vi "OSSCAR_v3_BM.vi"() -> ()   [LabVIEW 2021]
uses:
  SubVIs/Plot_trap_heating_global_BM.vi
  SubVIs/OSSCAR_stop_global_BM.vi
  SubVIs/DMSO-related/Temp_global_BM.vi
panel:
  out "Current Analyte:":string="DMS"
  in  "N std pt.s":i32=6
  in  "Mode Selection":T1(ring)
  in  "Standalone Function":T2(ring)
  out "Reduction Countdown (min)":dbl format="%.2g"
  out "Hydrolysis Countdown (min)":dbl format="%.2g"
  out "Sparge Countdown (min)":dbl format="%.2g"
  out "Elution Countdown (min)":dbl format="%.2f"
  out "Hydrolysis Progress Bar":u8(slide)=100 scale=0.0..100.0
  out "Reduction Progress Bar":u8(slide)=100 scale=0.0..100.0
  out "Elution Progress Bar":u8(slide)=100 scale=0.0..100.0
  out "Sparging Progress Bar":u8(slide)=100 scale=0.0..100.0
  in  "Analysis Type":T3(ring)
  in  "Tab Control":T4(tab)
  in  "Metadata":T5={"Local save location:"="C:\\Users\\LabPC1\\OneDrive\\Desktop\\OSSCAR_metadata\\Test_metadata", "Cruise ID"="LaPerouse", "Sampling Timestamp"="2023-07-19 15:23:13", "Elution Timestamp"="2023-07-19 15:29:12", "GPS_Latitude"=-999.0, "GPS_Longitude"=-999.0, "DMS_std_conc"=0.0, "DMSP_std_conc"=0.0, "DMSO_std_conc"=0.0, "Std_index"=0.0, "Initial Trap Temp (oC)"=30.0, "Max Trap Temp (oC)"=304.0, "Final Trap Temp (oC)"=30.0, "Flow Rate (mL/min)"=0.0, "Comment"="", "GPS_Minute"=-999.0, "GPS_Day"=-999.0, "GPS_jd"=-999.0, "GPS_Hour"=-999.0, "GPS_Second"=-999.0, "GPS Baud"=4800.0, "COM Port (GPS)"="COM10", "Use GPS?"=FALSE, "Format Date"="%d-%d-%d"} {"GPS_Latitude" format="%_4g"; "GPS_Longitude" format="%_4g"; "GPS_jd" format="%_5g"; "Std_index" format="%.2g"; "DMSO_std_conc" format="%.2f"; "DMSP_std_conc" format="%.2f"; "DMS_std_conc" format="%.2f"}
  in  "Sample Params":T6={"DMS Sparge Time (min)"=7.0, "Elution Time (min)"=1.5, "COM port (16 Pos. Valve)"="COM10", "Trap Heating Time (ms)"=500.0, "COM Port (DC Power)"="COM5", "COM Port (Runze)"="COM3", "sample volume"=10.0, "DMSO red. Sparge Time  (min)"=32.0, "DMSO Red. Duration (min)"=30.0, "Bypass sample handling (debugging)"=FALSE, "Reverse Reduction?"=FALSE, "Voltage (V)"="4.0", "DMSP Hydrolysis Time (min)"=13.0}
  in  "Constants":T7={"step to ml"=1920.0, "BoardNum"=0, "PosA BitNum"=1, "PosB BitNum"=2, "Heat Pulse Delay (ms)"=1000.0, "Heating Iterations"=6, "N rinses"=2, "Dissolution Time (s)"=120, "SpargeBit"=0, "Extra Milli-Q (ml)"=2.0, "Valco Port Number"=6, "BitNum (Thermocouple)"=1, "Total Vol. (mL)"=10.0, "N syringe rinses"=2, "NaOH Vol (ml)"=2.0, "FanBit"=4}
  in  "Pump Parameters":T8={"Speed 1"="100", "Speed 2"="250", "Speed 3"="350", "Speed 4"="250", "UW/Sample"="5", "Sparge"="2", "Std"="4", "Waste"="15", "Air"="14", "Milli-Q"="1", "H2SO4"="6", "NaOH"="3", "Catalyst"="7", "Cell (H+ side)"="8", "Cell (sample side)"="9", "NaCl"="11"}
  out "Current Temp:":i32=29
  out "Trap Heating":cluster{"Y":dbl[], "Y":dbl[]}[](graph)
  # "OSSCAR DMS/O/P Program"
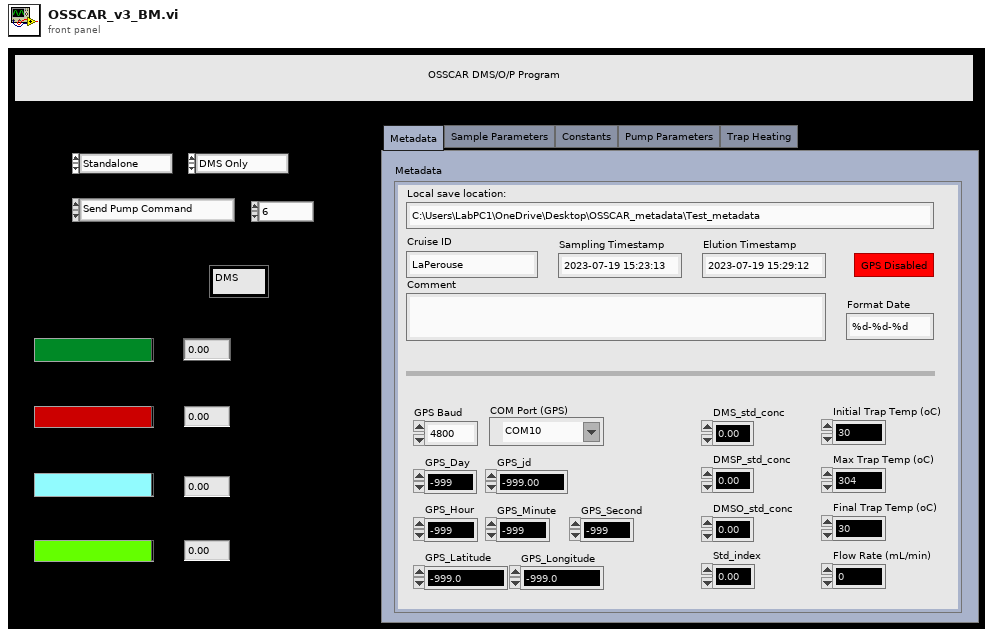
[diagram p1: front panel]
types:
  T1 = enum16{"Standalone", "Analysis", "Standard Curve", "Point Std"}
  T2 = enum16{"Send Pump Command", "Condition Trap", "Control Fan", "Control Sparger", "Load/Inject Trap", "Switch Flow Path", "Control cell DC power", "Rinse Sparge Chamber", "Rinse Cell"}
  T3 = enum16{"DMS Only", "DMS/O", "DMS/P", "DMS/O/P", "DMSO Only"}
  T4 = enum32{"Metadata", "Sample Parameters", "Constants", "Pump Parameters", "Trap Heating"}
  T5 = cluster{"Local save location:":string, "Cruise ID":string, "Sampling Timestamp":string, "Elution Timestamp":string, "GPS_Latitude":dbl, "GPS_Longitude":dbl, "DMS_std_conc":dbl, "DMSP_std_conc":dbl, "DMSO_std_conc":dbl, "Std_index":dbl, "Initial Trap Temp (oC)":dbl, "Max Trap Temp (oC)":dbl, "Final Trap Temp (oC)":dbl, "Flow Rate (mL/min)":dbl, "Comment":string, "GPS_Minute":dbl, "GPS_Day":dbl, "GPS_jd":dbl, "GPS_Hour":dbl, "GPS_Second":dbl, "GPS Baud":dbl, "COM Port (GPS)":refnum<visa-resource-name>, "Use GPS?":bool, "Format Date":string}
  T6 = cluster{"DMS Sparge Time (min)":dbl, "Elution Time (min)":dbl, "COM port (16 Pos. Valve)":refnum<visa-resource-name>, "Trap Heating Time (ms)":dbl, "COM Port (DC Power)":refnum<visa-resource-name>, "COM Port (Runze)":refnum<visa-resource-name>, "sample volume":dbl, "DMSO red. Sparge Time  (min)":dbl, "DMSO Red. Duration (min)":dbl, "Bypass sample handling (debugging)":bool, "Reverse Reduction?":bool, "Voltage (V)":string, "DMSP Hydrolysis Time (min)":dbl}
  T7 = cluster{"step to ml":dbl, "BoardNum":u32, "PosA BitNum":u32, "PosB BitNum":u32, "Heat Pulse Delay (ms)":dbl, "Heating Iterations":i32, "N rinses":i32, "Dissolution Time (s)":u32, "SpargeBit":u32, "Extra Milli-Q (ml)":dbl, "Valco Port Number":i32, "BitNum (Thermocouple)":u32, "Total Vol. (mL)":dbl, "N syringe rinses":i32, "NaOH Vol (ml)":dbl, "FanBit":u32}
  T8 = cluster{"Speed 1":string, "Speed 2":string, "Speed 3":string, "Speed 4":string, "UW/Sample":string, "Sparge":string, "Std":string, "Waste":string, "Air":string, "Milli-Q":string, "H2SO4":string, "NaOH":string, "Catalyst":string, "Cell (H+ side)":string, "Cell (sample side)":string, "NaCl":string}
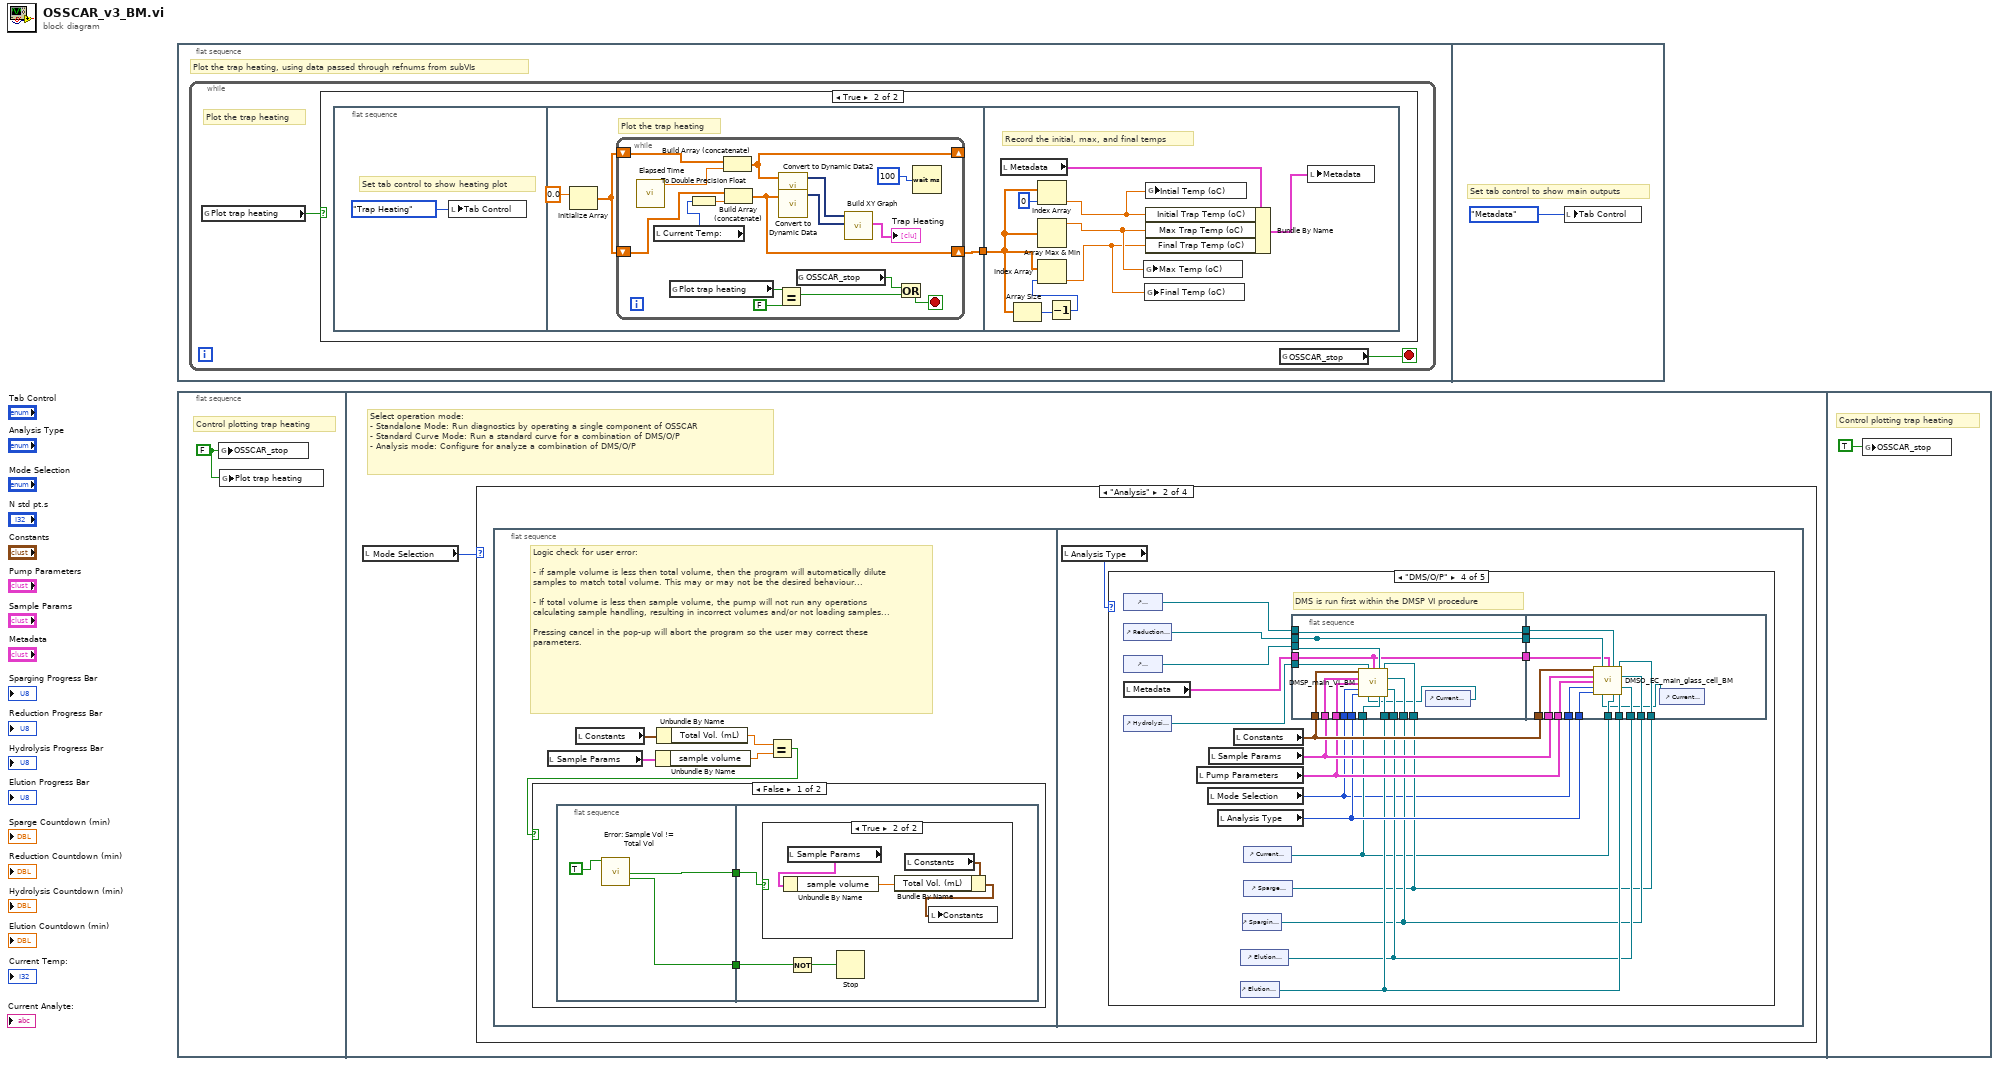
[diagram p0: block diagram]
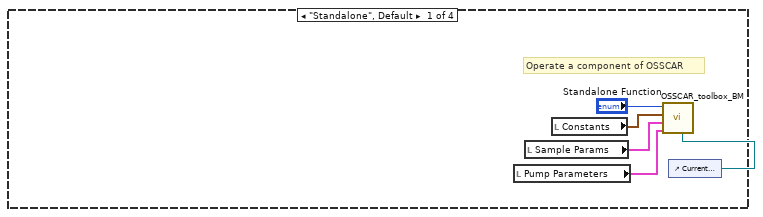
[diagram p3: hidden frame]
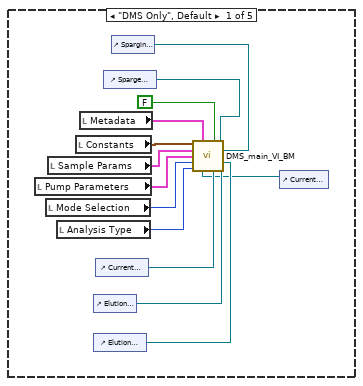
[diagram p6: hidden frame]
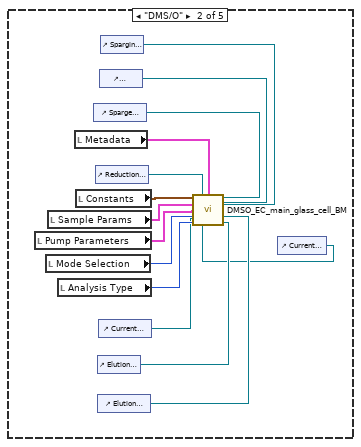
[diagram p7: hidden frame]
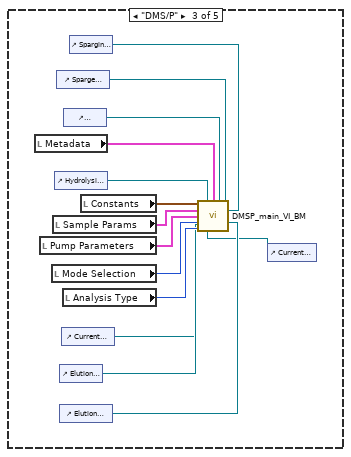
[diagram p8: hidden frame]
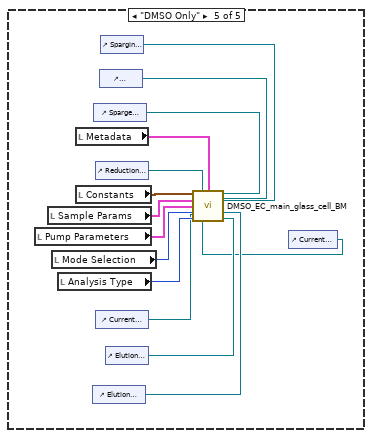
[diagram p9: hidden frame]
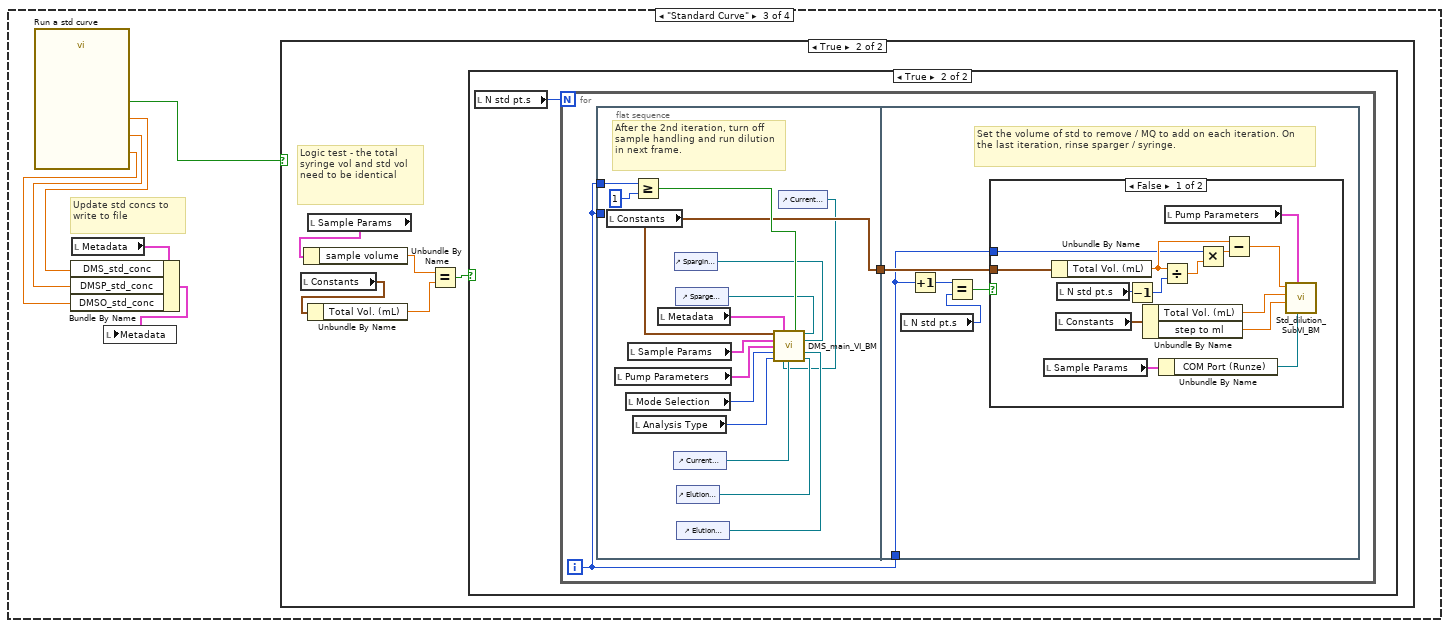
[diagram p10: hidden frame]
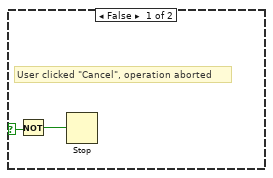
[diagram p11: hidden frame]
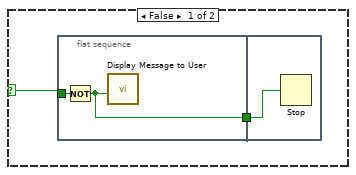
[diagram p12: hidden frame]
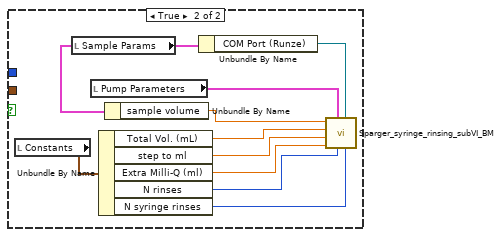
[diagram p13: hidden frame]
diagram:
  n1 = flat-sequence {
    frame #0 {
      # "Plot the trap heating, using data passed through refnums from subVIs"
      n2 = while {
        stop <- w2 stop-if-true
        # "Plot the trap heating"
        n3 = global read "Plot_trap_heating_global_BM.vi" "Plot trap heating"() -> (w1:bool)
        n4 = case shown="True" w1 {
          frame False {
            # "Do nothing when the trap isn't heating"
          }
          frame True {
            n5 = flat-sequence {
              tunnel: [w7] -> w3
              tunnel: w3 -> [w27]
              frame #0 {
                # "Set tab control to show heating plot"
                n6 = local write "Tab Control"(T4."Trap Heating" ("Tab Control 2")) -> ()
              }
              frame #1 {
                # "Plot the trap heating"
                n7 = Initialize Array(0.0 ("element")) -> (w5:dbl[])  [unwired: 1 in]
                n8 = while {
                  shift-right: [w14] -> w7
                  shift-left: w5 -> [w16]
                  shift-right: [w9] -> _
                  shift-left: w5 -> [w11]
                  stop <- w21 stop-if-true
                  n9 = call "Elapsed Time"() -> ("Elapsed Time (s)"=w12:dbl)  [unwired: 12 in, 7 out]
                  n10 = local read "Current Temp:"() -> (w23:i32)
                  n11 = global read "Plot_trap_heating_global_BM.vi" "Plot trap heating"() -> (w20:bool)
                  n12 = To Double Precision Float(number=w23) -> (double precision float=w17:dbl)
                  n13 = Build Array (concatenate)(w11, w12) -> (w9:dbl[])
                  n14 = Build Array (concatenate)(w16, w17) -> (w14:dbl[])
                  n15 = Equal?(x=w20, y=FALSE) -> (x = y?=w18:bool)
                  n16 = call "Convert to Dynamic Data2"("Array"=w9) -> ("Dynamic Data Type"=w10:dynamicdata)  [unwired: 3 in]
                  n17 = call "Convert to Dynamic Data"("Array"=w14) -> ("Dynamic Data Type"=w13:dynamicdata)  [unwired: 3 in]
                  n18 = global read "OSSCAR_stop_global_BM.vi" "OSSCAR_stop"() -> (w22:bool)
                  n19 = call "Build XY Graph"("Y Input"=w13, "X Input"=w10) -> ("XY Graph"=→"Trap Heating":cluster{"X":dbl[], "Y":dbl[]}[])  [unwired: 8 in, 1 out]
                  n20 = Or(x=w22, y=w18) -> (x .or. y?=w21:bool)
                  n21 = Wait (ms)(milliseconds to wait=u32 100) -> ()  [unwired: 1 out]
                }
              }
              frame #2 {
                # "Record the initial, max, and final temps"
                n22 = local read "Metadata"() -> (w32:T5)
                n23 = Array Size(array=w27) -> (size(s)=w29:i32)
                n24 = Index Array(array=w27, index=0) -> (element=w26:dbl)
                n25 = Array Max & Min(array=w27) -> (max value=w25:dbl)  [unwired: 3 out]
                n26 = Decrement(x=w29) -> (x-1=w28:i32)
                n27 = Index Array(array=w27, index=w28) -> (element=w24:dbl)
                n28 = global write "Temp_global_BM.vi" "Max Temp (oC)"(w25) -> ()
                n29 = global write "Temp_global_BM.vi" "Final Temp (oC)"(w24) -> ()
                n30 = global write "Temp_global_BM.vi" "Intial Temp (oC)"(w26) -> ()
                n31 = Bundle By Name(cluster=w32, "Initial Trap Temp (oC)"=w26, "Max Trap Temp (oC)"=w25, "Final Trap Temp (oC)"=w24) -> (w30:T5)
                n32 = local write "Metadata"(w30) -> ()
              }
            }
          }
        }
        n33 = global read "OSSCAR_stop_global_BM.vi" "OSSCAR_stop"() -> (w2:bool)
      }
    }
    frame #1 {
      # "Set tab control to show main outputs"
      n34 = local write "Tab Control"(T4."Metadata" ("Tab Control 2")) -> ()
    }
  }
  n35 = flat-sequence {
    frame #0 {
      w34 = FALSE ("OSSCAR_stop")
      # "Control plotting trap heating"
      n36 = global write "OSSCAR_stop_global_BM.vi" "OSSCAR_stop"(w34) -> ()
      n37 = global write "Plot_trap_heating_global_BM.vi" "Plot trap heating"(w34) -> ()
    }
    frame #1 {
      # "Select operation mode:\n- Standalone Mode: Run diagnostics by operating a single component of OSSCAR\n- Standard Curve Mode: Run a standard curve for a combination of DMS/O/P\n- Analysis mode: Configure for analyze a combination of DMS/O/P"
      n38 = local read "Mode Selection"() -> (w35:T1)
      n39 = case shown="\"Analysis\"" w35 {
        frame "Standalone", Default {
          # "Operate a component of OSSCAR"
          n40 = local read "Pump Parameters"() -> (w36:T8)
          n41 = local read "Sample Params"() -> (w37:T6)
          n42 = local read "Constants"() -> (w38:T7)
          n43 = control-ref of="Current Temp:"() -> (w39:refnum<vi>)
          n44 = call "OSSCAR_toolbox_BM.vi"("Temp Refnum"=w39, "Pump Parameters"=w36, "Sample Params"=w37, "Constants"=w38, "Function"="Standalone Function") -> ()  [unwired: 7 in]
        }
        frame "Analysis" {
          n45 = flat-sequence {
            frame #0 {
              # "Logic check for user error:\n\n- if sample volume is less then total volume, then the program will automatically dilute samples to match total volume. This may or may not be the desired behaviour...\n\n- If total volume is less then sample volume, the pump will not run any operations calculating sample handling, resulting in incorrect volumes and/or not loading samples...\n\nPressing cancel in the pop-up will abort the program so the user may correct these parameters."
              n46 = local read "Sample Params"() -> (w45:T6)
              n47 = local read "Constants"() -> (w44:T7)
              n48 = Unbundle By Name(w45) -> ("sample volume"=w43:dbl)
              n49 = Unbundle By Name(w44) -> ("Total Vol. (mL)"=w42:dbl)
              n50 = Equal?(x=w42, y=w43) -> (x = y?=w41:bool)
              n51 = case shown="False" w41 {
                frame False {
                  n52 = flat-sequence {
                    tunnel: [w50] -> w47
                    tunnel: [w49] -> w46
                    tunnel: w47 -> [w53]
                    tunnel: w46 -> [w51]
                    frame #0 {
                      n53 = call "Error: Sample Vol != Total Vol"("Enable"=TRUE) -> ("Make Total Vol = Sample Vol?"=w49:bool, "Proceed"=w50:bool)  [unwired: 16 in, 1 out]
                    }
                    frame #1 {
                      n54 = case shown="True" w51 {
                        frame False {
                          # "User indicated sample vol should not equal total vol, continue to analysis."
                        }
                        frame True {
                          n55 = local read "Sample Params"() -> (w57:T6)
                          n56 = Unbundle By Name(w57) -> ("sample volume"=w54:dbl)
                          n57 = local read "Constants"() -> (w56:T7)
                          n58 = Bundle By Name(cluster=w56, "Total Vol. (mL)"=w54) -> (w55:T7)
                          n59 = local write "Constants"(w55) -> ()
                        }
                      }
                      n60 = Not(x=w53) -> (.not. x?=w52:bool)
                      n61 = Stop(stop? (T)=w52) -> ()
                    }
                  }
                }
                frame True {
                  # "Else: carry on, nothing to see here..."
                }
              }
            }
            frame #1 {
              n62 = local read "Analysis Type"() -> (w58:T3)
              n63 = case shown="\"DMS/O/P\"" w58 {
                frame "DMS Only", Default {
                  n64 = local read "Pump Parameters"() -> (w70:T8)
                  n65 = local read "Mode Selection"() -> (w59:T1)
                  n66 = local read "Sample Params"() -> (w71:T6)
                  n67 = local read "Analysis Type"() -> (w69:T3)
                  n68 = local read "Constants"() -> (w62:T7)
                  n69 = local read "Metadata"() -> (w61:T5)
                  n70 = control-ref of="Elution Progress Bar"() -> (w64:refnum<vi>)
                  n71 = control-ref of="Elution Countdown (min)"() -> (w65:refnum<vi>)
                  n72 = control-ref of="Current Temp:"() -> (w63:refnum<vi>)
                  n73 = control-ref of="Sparge Countdown (min)"() -> (w67:refnum<vi>)
                  n74 = control-ref of="Sparging Progress Bar"() -> (w66:refnum<vi>)
                  n75 = control-ref of="Current Analyte:"() -> (w60:refnum<vi>)
                  n76 = call "DMS_main_VI_BM.vi"("Constants"=w62, "Metadata"=w61, "Skip sample handling"=FALSE, "Sparging Countdown Timer Refnum"=w67, "Sample Params"=w71, "Sparging Progress Bar Refnum"=w66, "Pump Parameters"=w70, "Mode Selection"=w59, "Elution Countdown Timer Refnum"=w65, "Analysis Type"=w69, "Current Analyte Refnum"=w60, "Temp Refnum"=w63, "Elution Progress Bar Refnum"=w64) -> ()  [unwired: 3 in]
                }
                frame "DMS/O" {
                  n77 = local read "Pump Parameters"() -> (w73:T8)
                  n78 = local read "Mode Selection"() -> (w72:T1)
                  n79 = local read "Sample Params"() -> (w84:T6)
                  n80 = local read "Analysis Type"() -> (w85:T3)
                  n81 = local read "Metadata"() -> (w75:T5)
                  n82 = local read "Constants"() -> (w76:T7)
                  n83 = control-ref of="Sparge Countdown (min)"() -> (w81:refnum<vi>)
                  n84 = control-ref of="Reduction Countdown (min)"() -> (w83:refnum<vi>)
                  n85 = control-ref of="Elution Progress Bar"() -> (w79:refnum<vi>)
                  n86 = control-ref of="Elution Countdown (min)"() -> (w78:refnum<vi>)
                  n87 = control-ref of="Current Temp:"() -> (w77:refnum<vi>)
                  n88 = control-ref of="Reduction Progress Bar"() -> (w82:refnum<vi>)
                  n89 = control-ref of="Sparging Progress Bar"() -> (w80:refnum<vi>)
                  n90 = control-ref of="Current Analyte:"() -> (w74:refnum<vi>)
                  n91 = call "DMSO_EC_main_glass_cell_BM.vi"("Constants"=w76, "Reduction Countdown Timer Refnum"=w83, "Metadata"=w75, "Reduction Progress Bar Refnum"=w82, "Sparging Countdown Timer Refnum"=w81, "Sample Params"=w84, "Sparging Progress Bar Refnum"=w80, "Pump Parameters"=w73, "Mode Selection"=w72, "Elution Countdown Timer Refnum"=w78, "Analysis Type"=w85, "Current Analyte Refnum"=w74, "Temp Refnum"=w77, "Elution Progress Bar Refnum"=w79) -> ()  [unwired: 2 in]
                }
                frame "DMS/P" {
                  n92 = local read "Metadata"() -> (w89:T5)
                  n93 = local read "Pump Parameters"() -> (w87:T8)
                  n94 = local read "Mode Selection"() -> (w86:T1)
                  n95 = local read "Sample Params"() -> (w98:T6)
                  n96 = control-ref of="Hydrolysis Countdown (min)"() -> (w94:refnum<vi>)
                  n97 = control-ref of="Sparge Countdown (min)"() -> (w92:refnum<vi>)
                  n98 = control-ref of="Elution Progress Bar"() -> (w96:refnum<vi>)
                  n99 = control-ref of="Elution Countdown (min)"() -> (w97:refnum<vi>)
                  n100 = control-ref of="Current Temp:"() -> (w91:refnum<vi>)
                  n101 = local read "Analysis Type"() -> (w99:T3)
                  n102 = control-ref of="Hydrolysis Progress Bar"() -> (w95:refnum<vi>)
                  n103 = control-ref of="Sparging Progress Bar"() -> (w93:refnum<vi>)
                  n104 = local read "Constants"() -> (w90:T7)
                  n105 = control-ref of="Current Analyte:"() -> (w88:refnum<vi>)
                  n106 = call "DMSP_main_VI_BM.vi"("Constants"=w90, "Hydrolysis Countdown Refnum"=w94, "Metadata"=w89, "Hydrolysis Progress Bar Refnum"=w95, "Sparge Countdown Timer Refnum"=w92, "Sample Params"=w98, "Sparging Progress Bar Refnum"=w93, "Pump Parameters"=w87, "Mode Selection"=w86, "Elution Countdown Timer Refnum"=w97, "Analysis Type"=w99, "Current Analyte Refnum"=w88, "Temp Refnum"=w91, "Elution Progress Bar Refnum"=w96) -> ()  [unwired: 2 in]
                }
                frame "DMS/O/P" {
                  # "DMS is run first within the DMSP VI procedure"
                  n107 = control-ref of="Reduction Progress Bar"() -> (w108:refnum<vi>)
                  n108 = control-ref of="Reduction Countdown (min)"() -> (w110:refnum<vi>)
                  n109 = control-ref of="Hydrolysis Progress Bar"() -> (w112:refnum<vi>)
                  n110 = local read "Metadata"() -> (w102:T5)
                  n111 = control-ref of="Hydrolysis Countdown (min)"() -> (w113:refnum<vi>)
                  n112 = local read "Pump Parameters"() -> (w115:T8)
                  n113 = local read "Mode Selection"() -> (w100:T1)
                  n114 = local read "Sample Params"() -> (w116:T6)
                  n115 = local read "Analysis Type"() -> (w114:T3)
                  n116 = local read "Constants"() -> (w117:T7)
                  n117 = control-ref of="Elution Countdown (min)"() -> (w106:refnum<vi>)
                  n118 = control-ref of="Elution Progress Bar"() -> (w107:refnum<vi>)
                  n119 = control-ref of="Sparging Progress Bar"() -> (w105:refnum<vi>)
                  n120 = control-ref of="Current Temp:"() -> (w103:refnum<vi>)
                  n121 = control-ref of="Sparge Countdown (min)"() -> (w104:refnum<vi>)
                  n122 = flat-sequence {
                    tunnel: w117 -> [w122]
                    tunnel: w116 -> [w133]
                    tunnel: w115 -> [w119]
                    tunnel: w114 -> [w132]
                    tunnel: w113 -> [w131]
                    tunnel: w112 -> [w130]
                    tunnel: [w129] -> _
                    tunnel: [w129] -> w111
                    tunnel: w110 -> [w129]
                    tunnel: w108 -> [w128]
                    tunnel: [w128] -> w109
                    tunnel: w104 -> [w127]
                    tunnel: w105 -> [w126]
                    tunnel: w106 -> [w125]
                    tunnel: w107 -> [w124]
                    tunnel: w103 -> [w123]
                    tunnel: w102 -> [w121]
                    tunnel: [w121] -> w101
                    tunnel: w100 -> [w118]
                    tunnel: w117 -> [w138]
                    tunnel: w116 -> [w147]
                    tunnel: w115 -> [w135]
                    tunnel: w114 -> [w146]
                    tunnel: w111 -> [w145]
                    tunnel: w109 -> [w144]
                    tunnel: w107 -> [w143]
                    tunnel: w106 -> [w142]
                    tunnel: w105 -> [w141]
                    tunnel: w104 -> [w140]
                    tunnel: w103 -> [w139]
                    tunnel: w101 -> [w137]
                    tunnel: w100 -> [w134]
                    frame #0 {
                      n123 = control-ref of="Current Analyte:"() -> (w120:refnum<vi>)
                      n124 = call "DMSP_main_VI_BM.vi"("Constants"=w122, "Hydrolysis Countdown Refnum"=w131, "Metadata"=w121, "Hydrolysis Progress Bar Refnum"=w130, "Sparge Countdown Timer Refnum"=w127, "Sample Params"=w133, "Sparging Progress Bar Refnum"=w126, "Pump Parameters"=w119, "Mode Selection"=w118, "Elution Countdown Timer Refnum"=w125, "Analysis Type"=w132, "Current Analyte Refnum"=w120, "Temp Refnum"=w123, "Elution Progress Bar Refnum"=w124) -> ()  [unwired: 2 in]
                    }
                    frame #1 {
                      n125 = control-ref of="Current Analyte:"() -> (w136:refnum<vi>)
                      n126 = call "DMSO_EC_main_glass_cell_BM.vi"("Constants"=w138, "Reduction Countdown Timer Refnum"=w145, "Metadata"=w137, "Reduction Progress Bar Refnum"=w144, "Sparging Countdown Timer Refnum"=w140, "Sample Params"=w147, "Sparging Progress Bar Refnum"=w141, "Pump Parameters"=w135, "Mode Selection"=w134, "Elution Countdown Timer Refnum"=w142, "Analysis Type"=w146, "Current Analyte Refnum"=w136, "Temp Refnum"=w139, "Elution Progress Bar Refnum"=w143) -> ()  [unwired: 2 in]
                    }
                  }
                }
                frame "DMSO Only" {
                  n127 = local read "Pump Parameters"() -> (w149:T8)
                  n128 = local read "Sample Params"() -> (w160:T6)
                  n129 = local read "Mode Selection"() -> (w148:T1)
                  n130 = local read "Analysis Type"() -> (w161:T3)
                  n131 = local read "Metadata"() -> (w151:T5)
                  n132 = local read "Constants"() -> (w152:T7)
                  n133 = control-ref of="Elution Countdown (min)"() -> (w154:refnum<vi>)
                  n134 = control-ref of="Sparge Countdown (min)"() -> (w157:refnum<vi>)
                  n135 = control-ref of="Reduction Countdown (min)"() -> (w159:refnum<vi>)
                  n136 = control-ref of="Current Temp:"() -> (w153:refnum<vi>)
                  n137 = control-ref of="Reduction Progress Bar"() -> (w158:refnum<vi>)
                  n138 = control-ref of="Sparging Progress Bar"() -> (w156:refnum<vi>)
                  n139 = control-ref of="Elution Progress Bar"() -> (w155:refnum<vi>)
                  n140 = control-ref of="Current Analyte:"() -> (w150:refnum<vi>)
                  n141 = call "DMSO_EC_main_glass_cell_BM.vi"("Constants"=w152, "Reduction Countdown Timer Refnum"=w159, "Metadata"=w151, "Reduction Progress Bar Refnum"=w158, "Sparging Countdown Timer Refnum"=w157, "Sample Params"=w160, "Sparging Progress Bar Refnum"=w156, "Pump Parameters"=w149, "Mode Selection"=w148, "Elution Countdown Timer Refnum"=w154, "Analysis Type"=w161, "Current Analyte Refnum"=w150, "Temp Refnum"=w153, "Elution Progress Bar Refnum"=w155) -> ()  [unwired: 2 in]
                }
              }
            }
          }
        }
        frame "Standard Curve" {
          # "Update std concs to write to file"
          n142 = call "Run a std curve"() -> ("DMSO std concentration"=w164:dbl, "DMSP std concentration"=w163:dbl, "DMS std concentration"=w162:dbl, "OK"=w167:bool)  [unwired: 15 in, 1 out]
          n143 = local read "Metadata"() -> (w166:T5)
          n144 = Bundle By Name(cluster=w166, "DMS_std_conc"=w162, "DMSP_std_conc"=w163, "DMSO_std_conc"=w164) -> (w165:T5)
          n145 = local write "Metadata"(w165) -> ()
          n146 = case shown="True" w167 {
            selector: w167 -> [w168 _]
            frame False {
              # "User clicked \"Cancel\", operation aborted"
              n147 = Not(x=w168) -> (.not. x?=w169:bool)
              n148 = Stop(stop? (T)=w169) -> ()
            }
            frame True {
              # "Logic test - the total syringe vol and std vol need to be identical"
              n149 = local read "Constants"() -> (w174:T7)
              n150 = local read "Sample Params"() -> (w173:T6)
              n151 = Unbundle By Name(w173) -> ("sample volume"=w170:dbl)
              n152 = Unbundle By Name(w174) -> ("Total Vol. (mL)"=w171:dbl)
              n153 = Equal?(x=w170, y=w171) -> (x = y?=w172:bool)
              n154 = case shown="True" w172 {
                selector: w172 -> [w175 _]
                frame False {
                  n155 = flat-sequence {
                    tunnel: w175 -> [w178]
                    tunnel: [w177] -> w176
                    tunnel: w176 -> [w179]
                    frame #0 {
                      n156 = Not(x=w178) -> (.not. x?=w177:bool)
                      n157 = call "Display Message to User"("Enable"=w177) -> ()  [unwired: 9 in, 2 out]
                    }
                    frame #1 {
                      n158 = Stop(stop? (T)=w179) -> ()
                    }
                  }
                }
                frame True {
                  n159 = local read "N std pt.s"() -> (w180:i32)
                  n160 = for {
                    N: w180 -> [_]
                    i -> [w181]
                    n161 = flat-sequence {
                      tunnel: w181 -> [w197]
                      tunnel: [w186] -> w182
                      tunnel: w181 -> [_]
                      tunnel: w181 -> [w200]
                      tunnel: w182 -> [w202]
                      frame #0 {
                        # "After the 2nd iteration, turn off sample handling and run dilution in next frame."
                        n162 = local read "Constants"() -> (w186:T7)
                        n163 = local read "Pump Parameters"() -> (w194:T8)
                        n164 = local read "Mode Selection"() -> (w183:T1)
                        n165 = local read "Sample Params"() -> (w193:T6)
                        n166 = Greater Or Equal?(x=w197, y=1) -> (x >= y?=w192:bool)
                        n167 = local read "Analysis Type"() -> (w195:T3)
                        n168 = local read "Metadata"() -> (w185:T5)
                        n169 = control-ref of="Current Temp:"() -> (w187:refnum<vi>)
                        n170 = control-ref of="Sparging Progress Bar"() -> (w190:refnum<vi>)
                        n171 = control-ref of="Sparge Countdown (min)"() -> (w191:refnum<vi>)
                        n172 = control-ref of="Elution Progress Bar"() -> (w188:refnum<vi>)
                        n173 = control-ref of="Elution Countdown (min)"() -> (w189:refnum<vi>)
                        n174 = control-ref of="Current Analyte:"() -> (w184:refnum<vi>)
                        n175 = call "DMS_main_VI_BM.vi"("Constants"=w186, "Metadata"=w185, "Skip sample handling"=w192, "Sparging Countdown Timer Refnum"=w191, "Sample Params"=w193, "Sparging Progress Bar Refnum"=w190, "Pump Parameters"=w194, "Mode Selection"=w183, "Elution Countdown Timer Refnum"=w189, "Analysis Type"=w195, "Current Analyte Refnum"=w184, "Temp Refnum"=w187, "Elution Progress Bar Refnum"=w188) -> ()  [unwired: 3 in]
                      }
                      frame #1 {
                        # "Set the volume of std to remove / MQ to add on each iteration. On the last iteration, rinse sparger / syringe."
                        n176 = local read "N std pt.s"() -> (w198:i32)
                        n177 = Increment(x=w200) -> (x+1=w199:i32)
                        n178 = Equal?(x=w199, y=w198) -> (x = y?=w201:bool)
                        n179 = case shown="False" w201 {
                          tunnel: w200 -> [w211 _]
                          tunnel: w202 -> [w210 _]
                          frame False {
                            n180 = local read "Sample Params"() -> (w205:T6)
                            n181 = Unbundle By Name(w210) -> ("Total Vol. (mL)"=w216:dbl)
                            n182 = local read "Constants"() -> (w208:T7)
                            n183 = local read "N std pt.s"() -> (w212:i32)
                            n184 = Decrement(x=w212) -> (x-1=w213:i32)
                            n185 = Unbundle By Name(w208) -> ("Total Vol. (mL)"=w207:dbl, "step to ml"=w206:dbl)
                            n186 = Unbundle By Name(w205) -> ("COM Port (Runze)"=w204:refnum<visa-resource-name>)
                            n187 = Divide(x=w216, y=w213) -> (x/y=w214:dbl)
                            n188 = local read "Pump Parameters"() -> (w203:T8)
                            n189 = Multiply(x=w211, y=w214) -> (x*y=w215:dbl)
                            n190 = Subtract(x=w216, y=w215) -> (x-y=w209:dbl)
                            n191 = call "Std_dilution_SubVI_BM.vi"("COM Port"=w204, "Pump Parameters"=w203, "step to ml"=w206, "Total Vol. (mL)"=w207, "Dilution Vol. (mL)"=w209) -> ()  [unwired: 7 in]
                          }
                          frame True {
                            n192 = local read "Constants"() -> (w217:T7)
                            n193 = local read "Sample Params"() -> (w218:T6)
                            n194 = local read "Pump Parameters"() -> (w220:T8)
                            n195 = Unbundle By Name(w217) -> ("Total Vol. (mL)"=w222:dbl, "step to ml"=w223:dbl, "Extra Milli-Q (ml)"=w224:dbl, "N rinses"=w225:i32, "N syringe rinses"=w226:i32)
                            n196 = Unbundle By Name(w218) -> ("sample volume"=w221:dbl)
                            n197 = Unbundle By Name(w218) -> ("COM Port (Runze)"=w219:refnum<visa-resource-name>)
                            n198 = call "Sparger_syringe_rinsing_subVI_BM.vi"("N syringe rinses"=w226, "COM Port"=w219, "N sparge rinses"=w225, "Pump Parameters"=w220, "Extra Milli-Q (ml)"=w224, "step to ml"=w223, "Total Vol. (mL)"=w222, "Sample Volume"=w221) -> ()  [unwired: 4 in]
                          }
                        }
                      }
                    }
                  }
                }
              }
            }
          }
        }
        frame "Point Std" {
        }
      }
    }
    frame #2 {
      # "Control plotting trap heating"
      n199 = global write "OSSCAR_stop_global_BM.vi" "OSSCAR_stop"(TRUE ("OSSCAR_stop")) -> ()
    }
  }
